vi "Turn off heating.vi"(8 "Все время процесса нанесения":dbl, 9 "Shift before":i32, 10 "Запуск процесса":bool, 11 "Текущее время":dbl) -> (0 "Boolean":bool, 1 "Shift after":i32, 5 "Время выхода до заданной температуры":dbl)   [LabVIEW 2012]
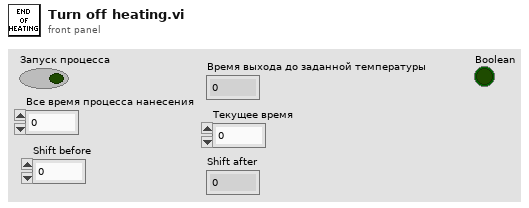
[diagram p1: front panel]
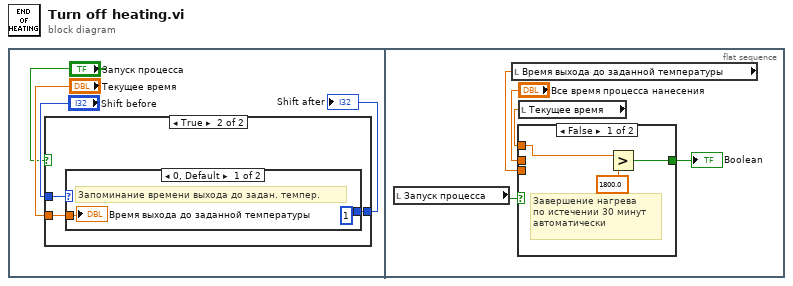
[diagram p0: block diagram]
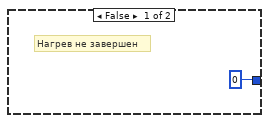
[diagram p2: hidden frame]
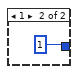
[diagram p3: hidden frame]
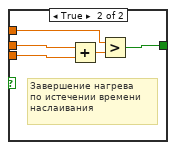
[diagram p4: hidden frame]
diagram:
  n1 = flat-sequence {
    frame #0 {
      n2 = case shown="True" "Запуск процесса" {
        tunnel: "Shift before" -> [_ w8]
        tunnel: "Текущее время" -> [_ w7]
        tunnel: [0 w6] -> w3
        frame False {
          # "Нагрев не завершен"
        }
        frame True {
          n3 = case shown="0, Default" w8 {
            tunnel: w7 -> [w9 _]
            tunnel: [1 1] -> w6
            frame 0, Default {
              # "Запоминание времени выхода до задан. темпер."
              "Время выхода до заданной температуры" <- w9
            }
            frame 1 {
            }
          }
        }
      }
      "Shift after" <- w3
    }
    frame #1 {
      n4 = local read "Запуск процесса"() -> (w12:bool)
      n5 = local read "Время выхода до заданной температуры"() -> (w14:dbl)
      n6 = local read "Текущее время"() -> (w13:dbl)
      n7 = case shown="False" w12 {
        tunnel: w14 -> [_ w22]
        tunnel: "Все время процесса нанесения" -> [_ w21]
        tunnel: [w18 w24] -> w15
        tunnel: w13 -> [w17 w20]
        frame False {
          # "Завершение нагрева\nпо истечении 30 минут\nавтоматически"
          n8 = Greater?(x=w17, y=1800.0) -> (0:w18:bool)
        }
        frame True {
          # "Завершение нагрева\nпо истечении времени\nнаслаивания"
          n9 = Add(x=w21, y=w22) -> (x+y=w23:dbl)
          n10 = Greater?(x=w20, y=w23) -> (0:w24:bool)
        }
      }
      "Boolean" <- w15
    }
  }
